vi "Vision_sRGBToCIE(Lab).vi"(7 "White Reference(D65)":cluster{"Xn":dbl, "Yn":dbl, "Zn":dbl}={"Xn"=0.950456, "Yn"=1.0, "Zn"=1.088754} {"Zn" format="%.6f"; "Yn" format="%.6f"; "Xn" format="%.6f"}, 8 "error in":errorcluster, 9 "Blue":u8, 10 "Green":u8, 11 "Red":u8) -> (0 "error out":errorcluster, 1 "b":dbl format="%.6f", 2 "a":dbl format="%.6f", 3 "L":dbl format="%.6f")   [LabVIEW 2013]
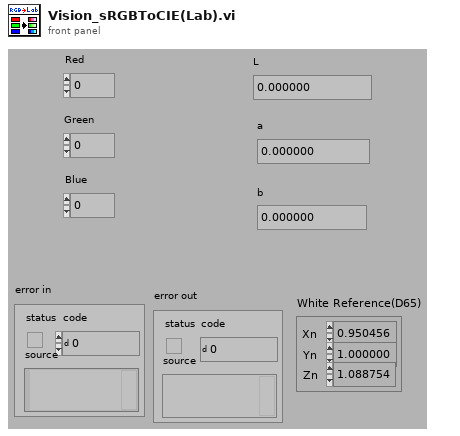
[diagram p1: front panel]
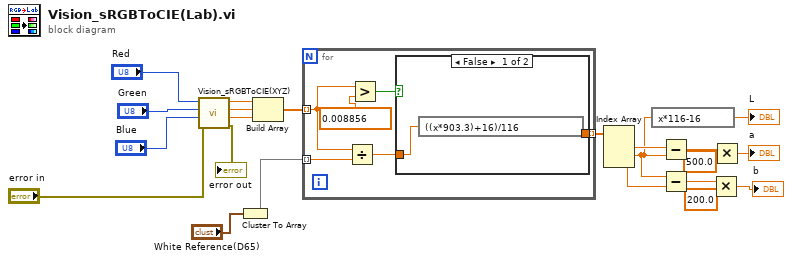
[diagram p0: block diagram]
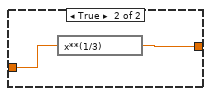
[diagram p2: hidden frame]
diagram:
  n1 = call "Vision_sRGBToCIE(XYZ).vi"("error in"="error in", "Blue"="Blue", "Green"="Green", "Red"="Red") -> ("error out"=→"error out":errorcluster, "Z"=w10:dbl, "Y"=w11:dbl, "X"=w12:dbl)  [unwired: 1 in, 3 out]
  n2 = Cluster To Array(cluster="White Reference(D65)") -> (array=w6:dbl[])
  n3 = Build Array(w12, w11, w10) -> (w22:dbl[])
  n4 = for {
    tunnel: w22 -> [w26] mode=indexing
    tunnel: w6 -> [w23] mode=indexing
    tunnel: [w24] -> w21 mode=indexing
    n5 = Divide(x=w26, y=w23) -> (x/y=w25:dbl)
    n6 = Greater?(x=w26, y=0.008856) -> (0:w27:bool)
    n7 = case shown="False" w27 {
      tunnel: w25 -> [w30 w32]
      tunnel: [w29 w31] -> w24
      frame False {
        n8 = expression code="((x*903.3)+16)/116"(w30) -> (w29:dbl)
      }
      frame True {
        n9 = expression code="x**(1/3)"(w32) -> (w31:dbl)
      }
    }
  }
  n10 = Index Array(array=w21) -> (element #1=w9:dbl, element #2=w8:dbl, element #3=w17:dbl)  [unwired: 3 in]
  n11 = expression code="x*116-16"(w8) -> (→"L":dbl)
  n12 = Subtract(x=w9, y=w8) -> (x-y=w18:dbl)
  n13 = Subtract(x=w8, y=w17) -> (x-y=w16:dbl)
  n14 = Multiply(x=w16, y=200.0) -> (x*y=→"b":dbl)
  n15 = Multiply(x=w18, y=500.0) -> (x*y=→"a":dbl)
